vi "Log Write.vi"(8 "error in (no error)":errorcluster, 11 "Log Message":T1) -> (0 "error out":errorcluster, 2 "Log Line":string, 3 "Log Message Out":T1)   [LabVIEW 2026, in "PXI_Common.lvlib"]
uses:
  PXI_Common.lvlib
  Types/Typedef/Log Message.ctl
  Types/Typedef/Log Message Levels.ctl
  Types/Enum/Bench Modules.ctl
  <vilib>/Utility/Data Type/NI_Data Type.lvlib
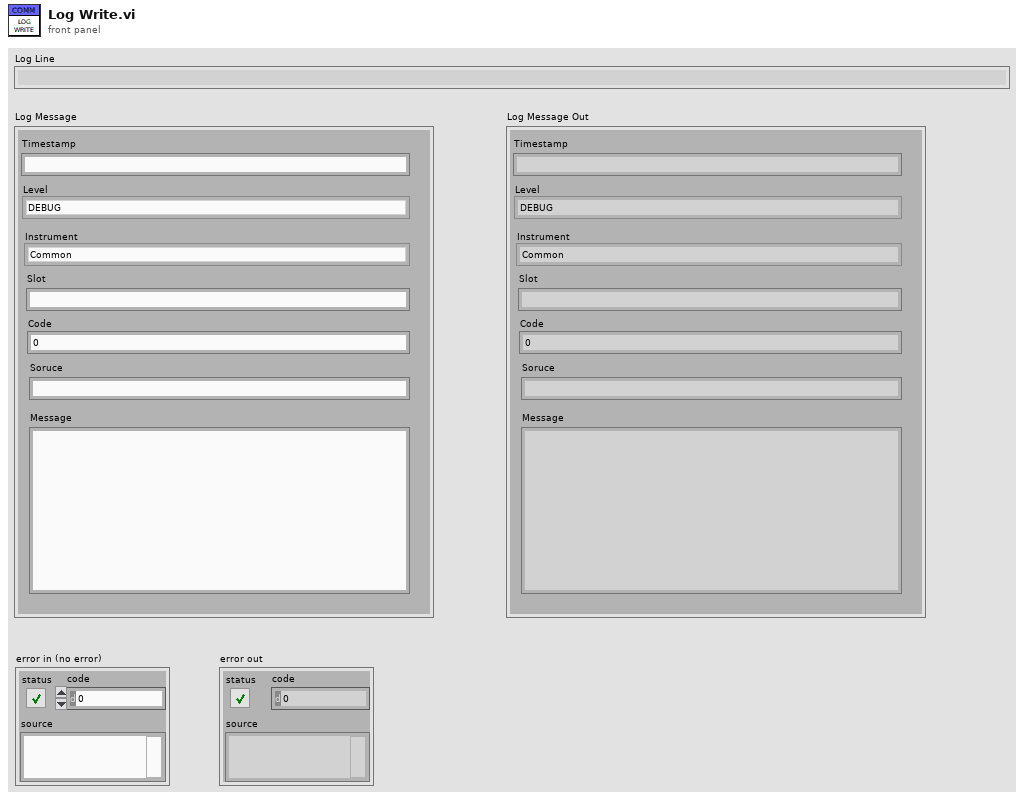
[diagram p1: front panel]
types:
  T1 = typedef "PXI_Common.lvlib/Log Message.ctl" = cluster{"Timestamp":string, "Level":T2, "Instrument":T3, "Slot":string, "Code":i32, "Soruce":string, "Message":string}
  T2 = typedef "PXI_Common.lvlib/Log Message Levels.ctl" = enum16{"DEBUG", "INFO", "WARNING", "ERROR"}
  T3 = typedef "PXI_Common.lvlib/Bench Modules.ctl" = enum16{"Common", "PXI4072", "PXI6259", "PXI6224", "PXI4130", "PXI8431"}
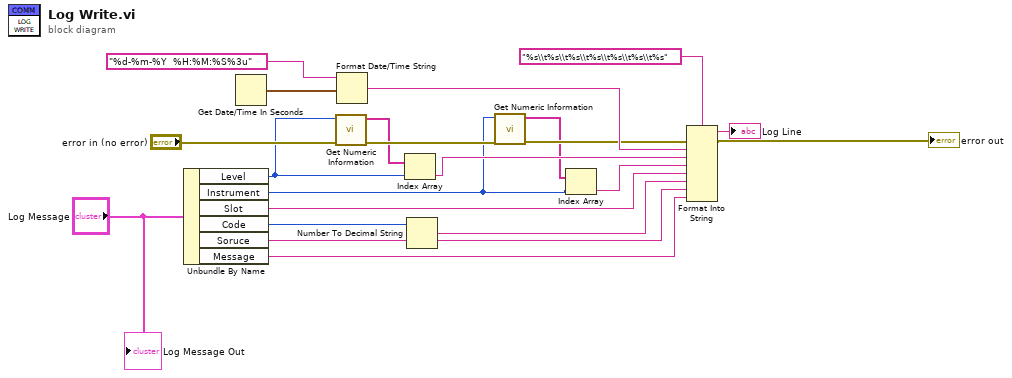
[diagram p0: block diagram]
diagram:
  n1 = Unbundle By Name("Log Message") -> ("Level"=w13:T2, "Instrument"=w9:T3, "Slot"=w7:string, "Code"=w6:i32, "Soruce"=w4:string, "Message"=w3:string)
  n2 = Get Date/Time In Seconds() -> (seconds since 1Jan1904=w20:timestamp)
  n3 = call <vilib>:"Get Numeric Information.vi"("error in (no error)"="error in (no error)", "variant"=w13) -> ("error out"=w14:errorcluster, "enum names"=w12:string[])  [unwired: 6 in, 2 out]
  n4 = Format Date/Time String(time format string (%c)="%d-%m-%Y  %H:%M:%S%3u", seconds (now)=w20) -> (date/time string=w17:string)  [unwired: 1 in]
  n5 = Index Array(array=w12, index=w13) -> (element=w11:string)
  n6 = Number To Decimal String(number=w6) -> (decimal integer string=w5:string)  [unwired: 1 in]
  n7 = call <vilib>:"Get Numeric Information.vi"("error in (no error)"=w14, "variant"=w9) -> ("error out"=w16:errorcluster, "enum names"=w10:string[])  [unwired: 6 in, 2 out]
  n8 = Index Array(array=w10, index=w9) -> (element=w8:string)
  n9 = Format Into String(format string="%s\\t%s\\t%s\\t%s\\t%s\\t%s\\t%s", error in=w16, w17, w11, w8, w7, w5, w4, w3) -> (resulting string=→"Log Line":string, error out=→"error out":errorcluster)  [unwired: 1 in]
  "Log Message Out" <- "Log Message"
